vi "Numero random con columna y fila.vi"() -> ()   [LabVIEW 2020]
panel:
  out "Array":dbl[][](array[numeric])
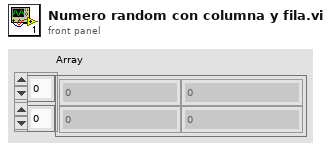
[diagram p1: front panel]
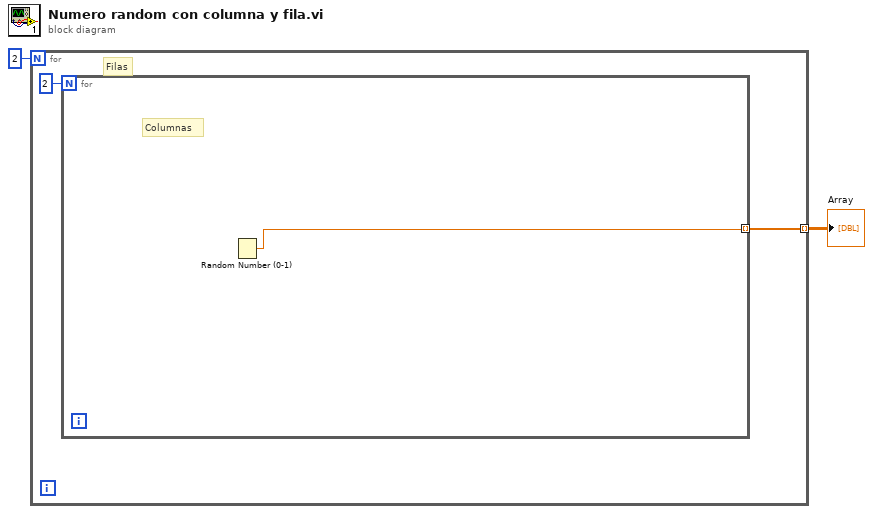
[diagram p0: block diagram]
diagram:
  n1 = for {
    N: 2 -> [_]
    tunnel: [w3] -> w1 mode=indexing
    # "Filas"
    n2 = for {
      N: 2 -> [_]
      tunnel: [w5] -> w3 mode=indexing
      # "Columnas"
      n3 = Random Number (0-1)() -> (number: 0 to 1=w5:dbl)
    }
  }
  "Array" <- w1
